vi "Create All Message Queues (host).vi"(8 "error in (no error)":errorcluster) -> (0 "error out":errorcluster, 3 "Message Queues":T1)   [LabVIEW 2018, in "Message Queue.lvlib"]
doc: "This VI creates and initializes all the message queues for your application. If your application requires more than one message queue, right-click the \"Message Queues\" constant above and select Open Type Def. Add the new Message Queue(s) to the type definition, then initialize them in this VI."
uses:
  Message Queue.lvlib
  All Message Queues (host).ctl
  Message Cluster (string).ctl
  Enqueue Message (string).vi
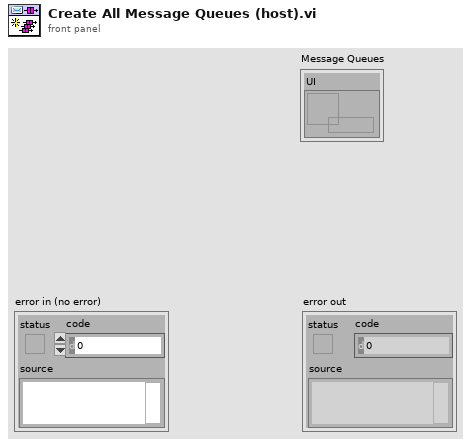
[diagram p1: front panel]
types:
  T1 = typedef "Message Queue.lvlib/All Message Queues (host).ctl" = cluster{"UI":refnum<queue>}
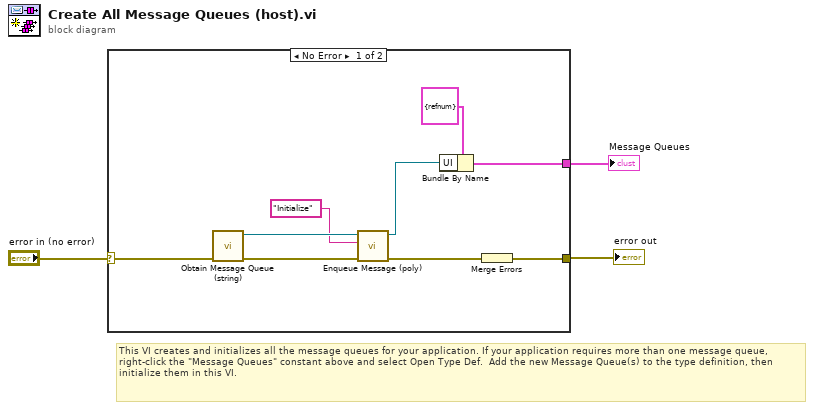
[diagram p0: block diagram]
diagram:
  # "This VI creates and initializes all the message queues for your application. If your application requires more than one message queue, right-click the \"Message Queues\" constant above and select Open Type Def.  Add the new Message Queue(s) to the type definition, then initialize them in this VI."
  n1 = case shown="No Error" "error in (no error)" {
    selector: "error in (no error)" -> [w7 w13]
    tunnel: [w11 w13] -> w3
    tunnel: [w12 _] -> w1
    frame No Error {
      n2 = call "Obtain Message Queue (string).vi"("error in (no error)"=w7) -> ("error out"=w6:errorcluster, "queue out"=w5:refnum<queue>)  [unwired: 9 in]
      n3 = call-poly "Enqueue Message (poly).vi"("error in (no error)"=w6, "Message"="Initialize", "Message Queue"=w5) -> ("error out"=w10:errorcluster, "dup Message Queue"=w9:refnum<queue>)  [unwired: 7 in]
      n4 = Bundle By Name(cluster=T1 {"UI"=refnum} ("Message Queues"), "UI"=w9) -> (w12:T1)
      n5 = Merge Errors(w10) -> (w11:errorcluster)
    }
    frame Error {
    }
  }
  "error out" <- w3
  "Message Queues" <- w1
